vi "MGI RWA Build Array Name.vi"(8 "Name In":string, 9 "Array":u32[](array[numeric]), 10 "Iteration":i32, 11 "Iterations":i32) -> (0 "Name Out":string)   [LabVIEW 2023]
doc: "This VI was created for use with the Read/Write Anything VIs. It builds the name used as the INI key for arrays which includes the array dimensions.\n\nAuthored by Robert C. Mortensen\nsupport@mooregoodideas.com\nwww.mooregoodideas.com\n\nCopyright (c) 2010, Moore Good Ideas, Inc.\n\nAll rights reserved.\n\nRedistribution and use in source and binary forms, with or without modification, are permitted provided that the following conditions are met:\n\n * Redistributions of source code must retain the above copyright notice, this list of conditions and the following disclaimer.\n * Redistributions in binary form must reproduce the above copyright notice, this list of conditions and the following disclaimer in the documentation and/or other materials provided with the distribution.\n * Neither the name of Moore Good Ideas, Inc. nor the names of its contributors may be used to endorse or promote products derived from this software without specific prior written permission.\n\nTHIS SOFTWARE IS PROVIDED BY THE COPYRIGHT HOLDERS AND CONTRIBUTORS \"AS IS\" AND ANY EXPRESS OR IMPLIED WARRANTIES, INCLUDING, BUT NOT LIMITED TO, THE IMPLIED WARRANTIES OF MERCHANTABILITY AND FITNESS FOR A PARTICULAR PURPOSE ARE DISCLAIMED. IN NO EVENT SHALL THE COPYRIGHT OWNER OR CONTRIBUTORS BE LIABLE FOR ANY DIRECT, INDIRECT, INCIDENTAL, SPECIAL, EXEMPLARY, OR CONSEQUENTIAL DAMAGES (INCLUDING, BUT NOT LIMITED TO, PROCUREMENT OF SUBSTITUTE GOODS OR SERVICES; LOSS OF USE, DATA, OR PROFITS; OR BUSINESS INTERRUPTION) HOWEVER CAUSED AND ON ANY THEORY OF LIABILITY, WHETHER IN CONTRACT, STRICT LIABILITY, OR TORT (INCLUDING NEGLIGENCE OR OTHERWISE) ARISING IN ANY WAY OUT OF THE USE OF THIS SOFTWARE, EVEN IF ADVISED OF THE POSSIBILITY OF SUCH DAMAGE."
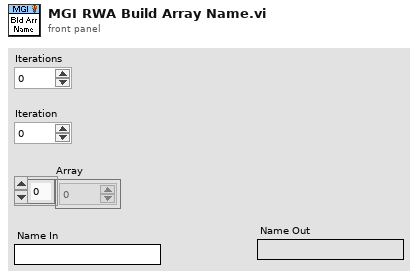
[diagram p1: front panel]
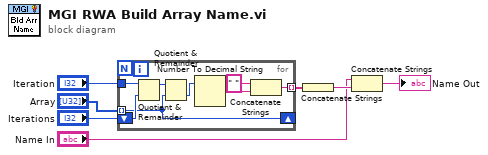
[diagram p0: block diagram]
diagram:
  n1 = for {
    tunnel: [w14] -> w4 mode=indexing
    tunnel: "Iteration" -> [w12]
    tunnel: "Array" -> [w9] mode=indexing
    shift-right: [w9] -> _
    shift-left: "Iterations" -> [w11]
    n2 = Quotient & Remainder(x=w12, y=w11) -> (x-y*floor(x/y)=w13:u32)  [unwired: 1 out]
    n3 = Quotient & Remainder(x=w13, y=w9) -> (floor(x/y)=w10:u32)  [unwired: 1 out]
    n4 = Number To Decimal String(number=w10) -> (decimal integer string=w15:string)  [unwired: 1 in]
    n5 = Concatenate Strings(" " ("string"), w15) -> (w14:string)
  }
  n6 = Concatenate Strings(w4) -> (w2:string)
  n7 = Concatenate Strings("Name In", w2) -> (→"Name Out":string)
